vi "Get Left Position.vi"(11 "drive in":refnum<class "drive.lvclass">) -> (2 "LPosition":dbl, 3 "drive out":refnum<class "drive.lvclass">)   [LabVIEW 2015, in "drive.lvclass"]
uses:
  drive.lvclass
  drive.lvclass/drive.ctl
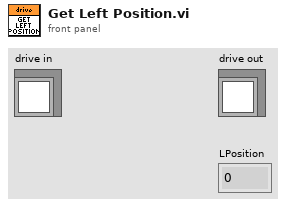
[diagram p1: front panel]
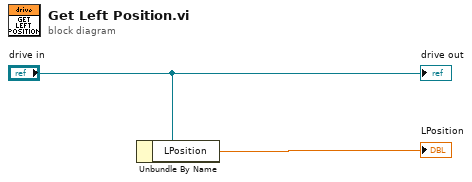
[diagram p0: block diagram]
diagram:
  n1 = Unbundle By Name("drive in") -> ("LPosition"=→"LPosition":dbl)
  "drive out" <- "drive in"
